vi "MT Generate MSK Synchronization Parameters (number array).vi"(0 "MSK system parameters":T1={"differential encoding enable"=enum."disable", "samples per symbol (16)"=16}, 1 "symbol rate (Hz)":dbl format="%.2f", 5 "sync numbers":i32[](array[numeric]) format="%.0x", 7 "bits per sync number":i32=32, 11 "error in (no error)":errorcluster, 12 "expected sync location (symbols)":i32=-1, 13 "sync location uncertainty (symbols)":i32=10, 14 "sync indent (symbols)":i32) -> (4 "MSK synchronization parameters":T2 {"sync sequence" format="%.2f"}, 15 "error out":errorcluster)   [LabVIEW 2020, in "niDMT.lvlib"]
doc: "This polymorphic instance generates synchronization parameters for MSK demodulation using a synchronization sequence defined by a <B>sync numbers</B> input array in which each number represents a group of bits."
uses:
  <vilib>/addons/Modulation/niDMT.lvlib
  <vilib>/addons/Modulation/niAMT.lvlib
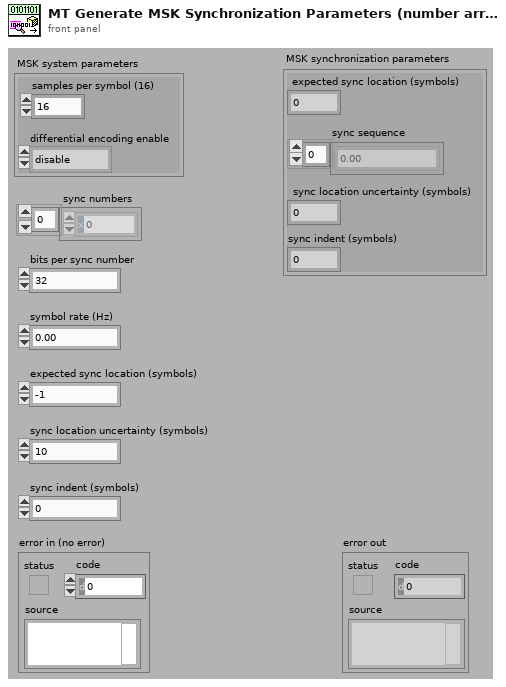
[diagram p1: front panel]
types:
  T1 = cluster{"differential encoding enable":enum16{"disable", "enable"}, "samples per symbol (16)":i32}
  T2 = cluster{"expected sync location (symbols)":i32, "sync sequence":cdb[], "sync location uncertainty (symbols)":i32, "sync indent (symbols)":i32}
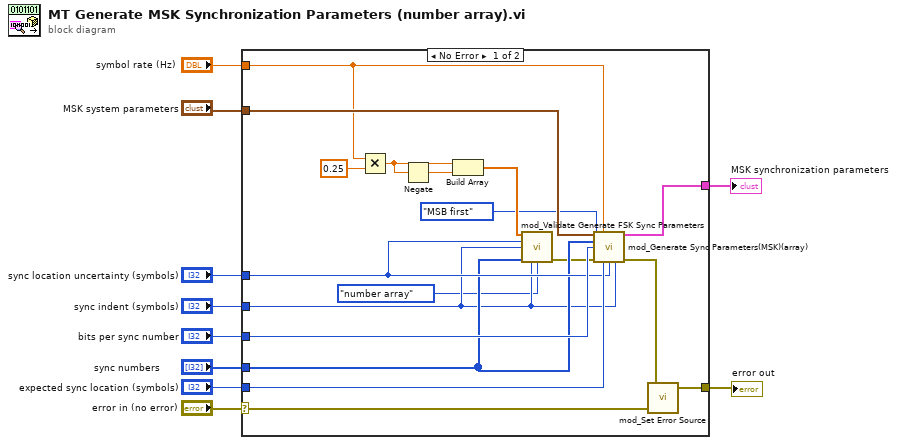
[diagram p0: block diagram]
diagram:
  n1 = case shown="No Error" "error in (no error)" {
    selector: "error in (no error)" -> [w25 w29]
    tunnel: "expected sync location (symbols)" -> [w24 _]
    tunnel: "sync location uncertainty (symbols)" -> [w16 _]
    tunnel: "sync indent (symbols)" -> [w13 _]
    tunnel: "sync numbers" -> [w15 _]
    tunnel: "bits per sync number" -> [w23 _]
    tunnel: [w28 w29] -> w4
    tunnel: "MSK system parameters" -> [w22 _]
    tunnel: "symbol rate (Hz)" -> [w21 _]
    tunnel: [w27 _] -> w1
    frame No Error {
      n2 = Multiply(x=w21, y=0.25) -> (x*y=w19:dbl)
      n3 = Negate(x=w19) -> (-x=w18:dbl)
      n4 = Build Array(w19, w18) -> (w17:dbl[])
      n5 = call <vilib>:"mod_Validate Generate FSK Sync Parameters.vi"("symbol map"=w17, "sync location uncertainty (symbols)"=w16, "sync indent (symbols)"=w13, "sync numbers"=w15, "number of bits (or) bits per number"=w13, "sync bits specification"=enum16{"bit array", "number array", "number"}."number array") -> ("error out"=w14:errorcluster)  [unwired: 1 in, 8 out]
      n6 = call <vilib>:"mod_Generate Sync Parameters(MSK)(array).vi"("MSK system parameters"=w22, "symbol rate (Hz)"=w21, "sync numbers"=w15, "bits per number"=w23, "bit order"=enum16{"MSB first", "LSB first"}."MSB first", "error in (no error)"=w14, "expected sync location (symbols)"=w24, "sync location uncertainty (symbols)"=w16, "sync indent (symbols)"=w13) -> ("MSK synchronization parameters"=w27:T2, "error out"=w26:errorcluster)  [unwired: 5 out]
      n7 = call <vilib>:"mod_Set Error Source.vi"("initial error in (no error)"=w25, "final error in (no error)"=w26) -> ("error out"=w28:errorcluster)  [unwired: 3 out]
    }
    frame Error {
    }
  }
  "MSK synchronization parameters" <- w1
  "error out" <- w4
